vi "Save LVClass.vi"(8 "error in (no error)":errorcluster, 11 "LVClassLibrary in":refnum<vi>) -> (0 "error out":errorcluster, 3 "LVClassLibrary out":refnum<vi>)   [LabVIEW 2019, in "VI Scripting Tools.lvlib"]
uses:
  VI Scripting Tools.lvlib
panel:
  in  "Path":path
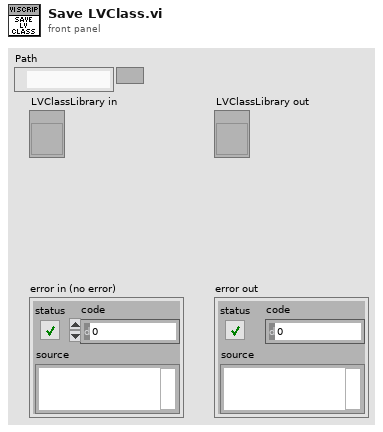
[diagram p1: front panel]
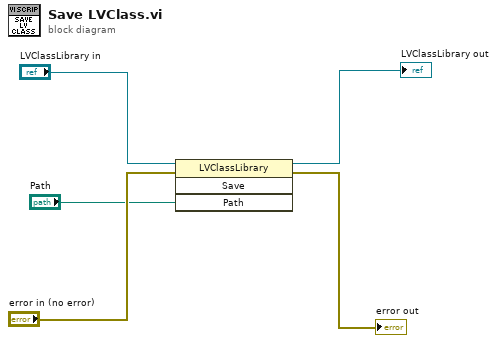
[diagram p0: block diagram]
diagram:
  n1 = invoke class="LVClassLibrary" method="Save"(reference="LVClassLibrary in", error in="error in (no error)", "Path"="Path") -> (reference out=→"LVClassLibrary out":refnum<vi>, error out=→"error out":errorcluster)  [unwired: 1 in, 2 out]
